vi "test_web_app.vi"() -> ()   [LabVIEW 2019]
panel:
  in  "Pause Button":bool
  in  "Knob":u64(knob)=511 scale=0.0..1000.0
  out "Number indicator":dbl
  in  "Stop Button":bool
  in  "Play Button":bool
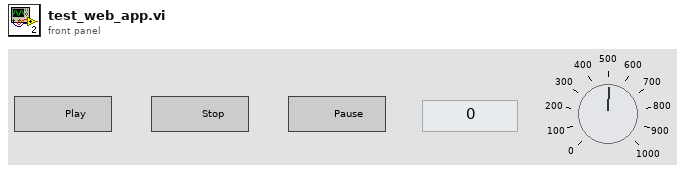
[diagram p1: front panel]
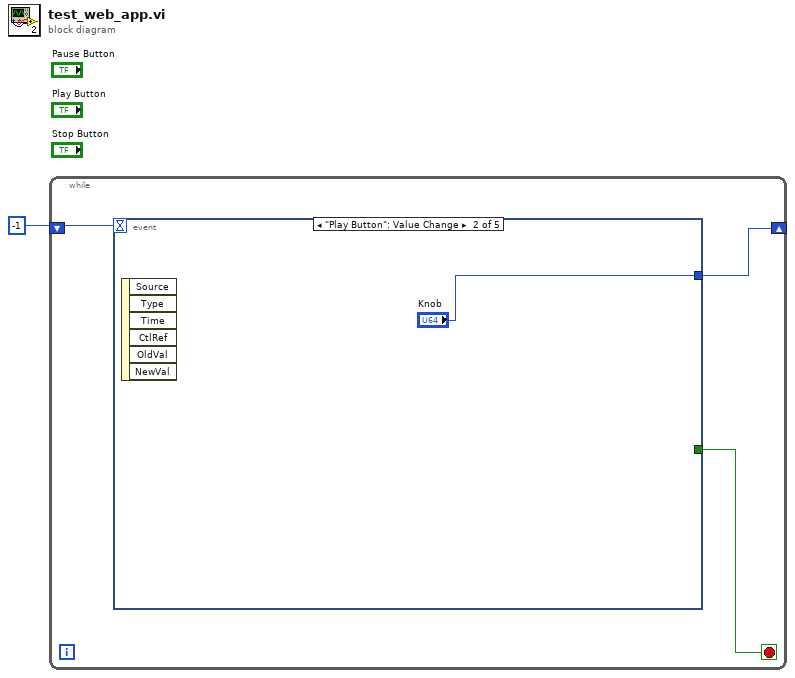
[diagram p0: block diagram]
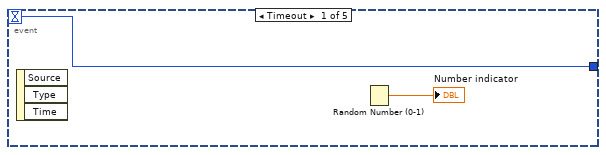
[diagram p2: hidden frame]
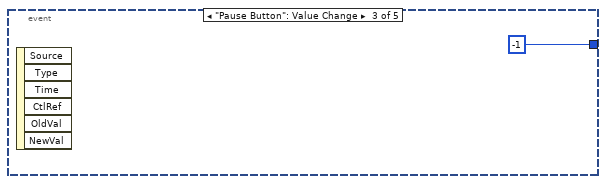
[diagram p3: hidden frame]
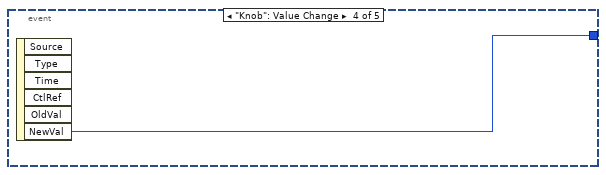
[diagram p4: hidden frame]
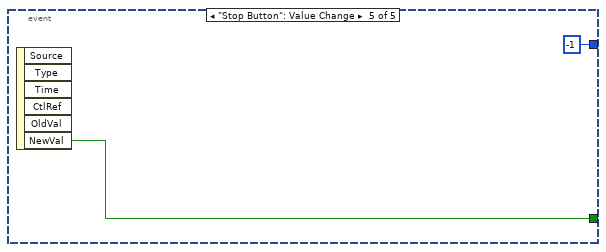
[diagram p5: hidden frame]
diagram:
  n1 = while {
    shift-right: [w2] -> _
    shift-left: -1 -> [w4]
    stop <- w3 stop-if-true
    n2 = event shown="[1] \"Play Button\": Value Change" {
      selector: _ -> [_ _ _ _ _]
      dyn-events: _ -> [_ _ _ _ _]
      timeout: w4 -> [w5 _ _ _ _]
      tunnel: [_ _ _ _ w11] -> w3
      tunnel: [w5 "Knob" -1 w9 -1 ("NewVal")] -> w2
      event Timeout {
        n3 = event-data() -> ()  [unwired: 1 in, 3 out]
        n4 = Random Number (0-1)() -> (number: 0 to 1=→"Number indicator":dbl)
      }
      event "Play Button": Value Change {
        n5 = event-data() -> ()  [unwired: 1 in, 6 out]
      }
      event "Pause Button": Value Change {
        n6 = event-data() -> ()  [unwired: 1 in, 6 out]
      }
      event "Knob": Value Change {
        n7 = event-data() -> ("NewVal"=w9:u64)  [unwired: 1 in, 5 out]
      }
      event "Stop Button": Value Change {
        n8 = event-data() -> ("NewVal"=w11:bool)  [unwired: 1 in, 5 out]
      }
    }
  }
